vi "easing_QuintOut.vi"(9 "distance":dbl, 10 "interval (10 ms)":dbl, 11 "time":dbl) -> (3 "current pos":dbl)   [LabVIEW 2023]
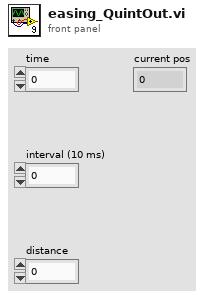
[diagram p1: front panel]
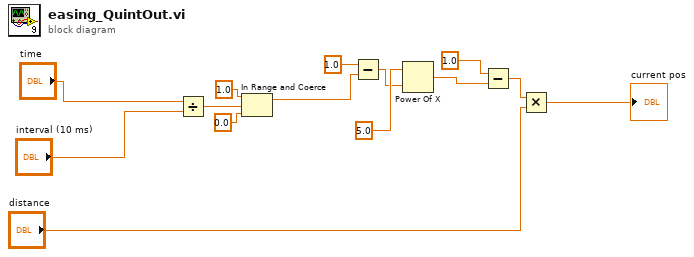
[diagram p0: block diagram]
diagram:
  n1 = Divide(x="time", y="interval (10 ms)") -> (x/y=w4:dbl)
  n2 = In Range and Coerce(upper limit=1.0, x=w4, lower limit=0.0 ("upper limit")) -> (coerced(x)=w1:dbl)  [unwired: 1 out]
  n3 = Subtract(x=1.0 ("y"), y=w1) -> (x-y=w7:dbl)
  n4 = Power Of X(1:w7, 2:5.0 ("y")) -> (0:w11:dbl)
  n5 = Subtract(x=1.0 ("y"), y=w11) -> (x-y=w12:dbl)
  n6 = Multiply(x=w12, y="distance") -> (x*y=→"current pos":dbl)
